vi "Wrapper_Destroy.vi"(2 "error in (no error)":errorcluster, 3 "Wrapper":u32) -> (0 "error out":errorcluster)   [LabVIEW 2012]
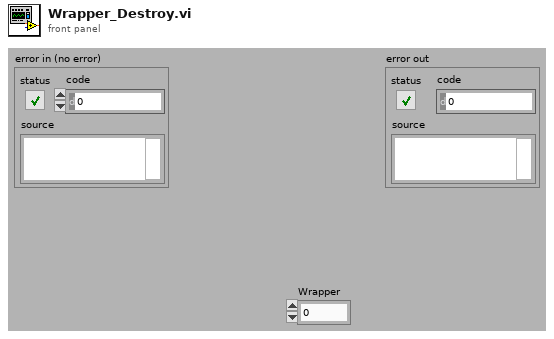
[diagram p1: front panel]
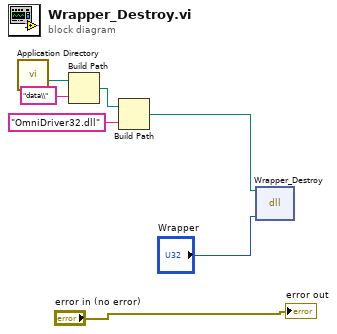
[diagram p0: block diagram]
diagram:
  n1 = call <vilib>:"Application Directory.vi"() -> ("Application Directory"=w6:path)
  n2 = Build Path(base path=w6, name or relative path="data\\") -> (appended path=w3:path)
  n3 = Build Path(base path=w3, name or relative path="OmniDriver32.dll") -> (appended path=w2:path)
  n4 = dll-call lib="D:/Software Development/EPI Development/BurnIn Testing/Instruments/Drivers/Ocean Optics/OOI_HOME/OmniDriver32.dll" fn="Wrapper_Destroy" label="Wrapper.Destroy"(path in=w2, "Wrapper"="Wrapper") -> ()  [unwired: 3 in, 3 out]
  "error out" <- "error in (no error)"
